vi "V_Gain.vi"(1 "Gain":T1) -> (0 "Gain (x)":dbl)   [LabVIEW 2019, in "Instrument.KH7008.lvclass"]
uses:
  Instrument.KH7008.lvclass
  typedefs/Gain-Enum.ctl
  faae6814-aeb4-44ba-9c01-adc0fb0891f6.vi
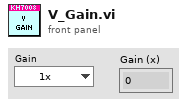
[diagram p1: front panel]
types:
  T1 = typedef "Instrument.KH7008.lvclass/Gain-Enum.ctl" = enum16{"1x", "10x", "100x", "1000x"}
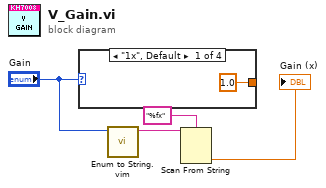
[diagram p0: block diagram]
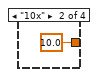
[diagram p2: hidden frame]
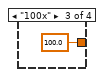
[diagram p3: hidden frame]
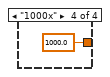
[diagram p4: hidden frame]
diagram:
  n1 = case shown="\"1x\", Default" "Gain" {
    tunnel: [1.0 ("y") 10.0 ("y") 100.0 ("y") 1000.0 ("y")] -> _
    frame "1x", Default {
    }
    frame "10x" {
    }
    frame "100x" {
    }
    frame "1000x" {
    }
  }
  n2 = call "Enum to String.vim"("Command"="Gain") -> ("Command"=w3:string)  [unwired: 9 in, 1 out]
  n3 = Scan From String(format string="%fx", input string=w3) -> (output 1=→"Gain (x)":dbl)  [unwired: 3 in, 3 out]
